vi "__parseReading.vi"(8 "error in (no error)":errorcluster, 9 "AlicatResponse":string="Y +014.56 +031.47 -00.001 -00.001 00.016    C2H6\r") -> (0 "error out":errorcluster, 1 "ParsedReading":T1={"ID"="", "Pressure"=13.55, "Temperature"=28.56, "Volumetric"=-1.9, "Mass"=-1.7, "SetPoint"=250.0, "Gas"="", "Total"=250.0} {"Total" format="%.2f"; "SetPoint" format="%.2f"; "Mass" format="%.2f"; "Volumetric" format="%.2f"; "Temperature" format="%.2f"; "Pressure" format="%.2f"})   [LabVIEW 2017]
uses:
  __Alicat SD_ReadingCluster.ctl
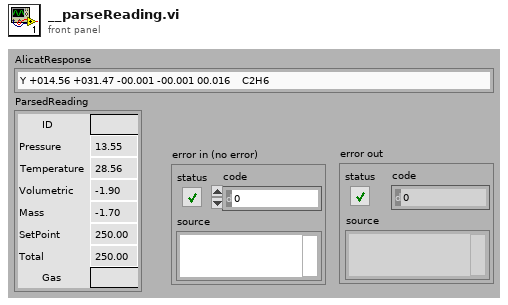
[diagram p1: front panel]
types:
  T1 = typedef "__Alicat SD_ReadingCluster.ctl" = cluster{"ID":string, "Pressure":sgl, "Temperature":sgl, "Volumetric":sgl, "Mass":sgl, "SetPoint":sgl, "Gas":string, "Total":sgl}
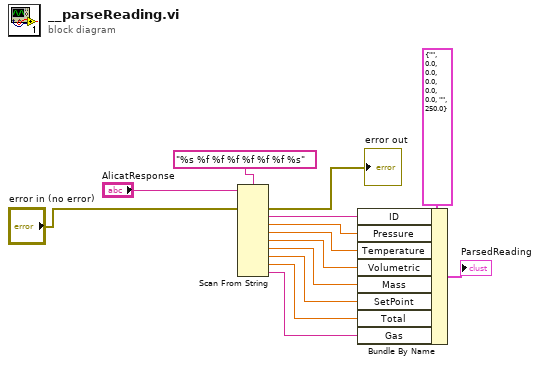
[diagram p0: block diagram]
diagram:
  n1 = Scan From String(format string="%s %f %f %f %f %f %f %s", input string="AlicatResponse", error in="error in (no error)") -> (error out=→"error out":errorcluster, output 1=w7:string, output 2=w4:dbl, output 3=w12:dbl, output 4=w11:dbl, output 5=w10:dbl, output 6=w9:dbl, output 7=w8:dbl, output 8=w1:string)  [unwired: 9 in, 2 out]
  n2 = Bundle By Name(cluster=T1 {"ID"="", "Pressure"=0.0, "Temperature"=0.0, "Volumetric"=0.0, "Mass"=0.0, "SetPoint"=0.0, "Gas"="", "Total"=250.0} ("ParsedReading"), "ID"=w7, "Pressure"=w4, "Temperature"=w12, "Volumetric"=w11, "Mass"=w10, "SetPoint"=w9, "Total"=w8, "Gas"=w1) -> (→"ParsedReading":T1)
